vi "VDD.vi"(8 "error in (no error)":errorcluster, 10 "Multimetru":refnum<visa-resource-name>="GPIB0::24::INSTR", 11 "SMU":refnum<visa-resource-name>="GPIB0::1::INSTR") -> (0 "error out":errorcluster, 1 "Histeresis":dbl, 2 "VDD_min_down":dbl, 3 "VDD_min_up":dbl)   [LabVIEW 2020]
uses:
  76adbe7d-9721-415f-b48f-f6746734e94a.vi
  a5dc711f-f3d3-4f32-829f-27d9f17150a9.vi
  eb78ffcd-5ce8-4557-ad43-e495a85b1885.vi
  a097896c-11b6-4113-a8a2-d510a1bfe5c9.vi
  204cda9c-a345-42f7-b798-14036ec7fdcd.vi
  845bcc2d-13a0-4ca5-84b0-81bd2e2c0ef6.vi
  9402af0b-bcf9-4b6a-9b28-d1ed00ce5349.vi
  <vilib>/Analysis/1siggen.llb/Ramp Pattern by Delta.vi
  Drivers/agilent_3446x_series/Agilent 3446X Series/Public/Data/Read (Single Point).vi
  Drivers/keithley_2450/Keithley 2450/Keithley 2450.lvlib
  Drivers/agilent_3446x_series/Agilent 3446X Series/Agilent 3446X Series.lvlib
  <vilib>/Analysis/NI_AALBase.lvlib
panel:
  in  "Tab Control":enum32{"Page 1", "Page 2"}(tab)
  out "IDD up":dbl
  out "noOfDevs out":u32=1
  out "VDD curent up":dbl
  out "VDD curent down":dbl
  out "noOfDevs out 2":u32=1
  out "IDD down":dbl
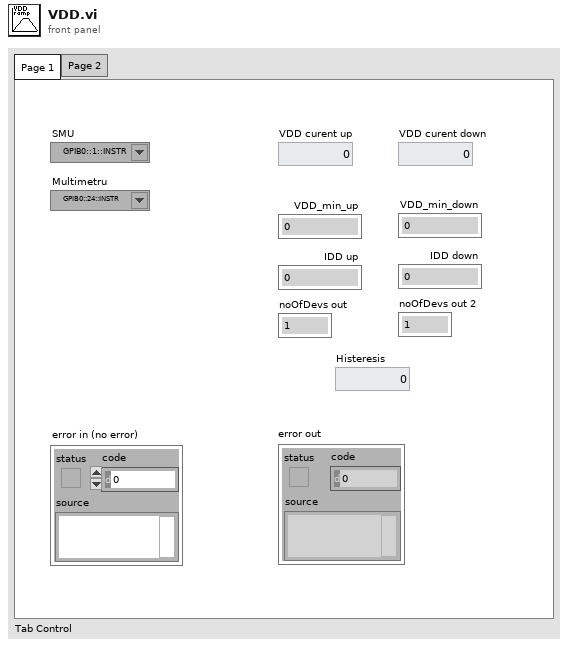
[diagram p1: front panel]
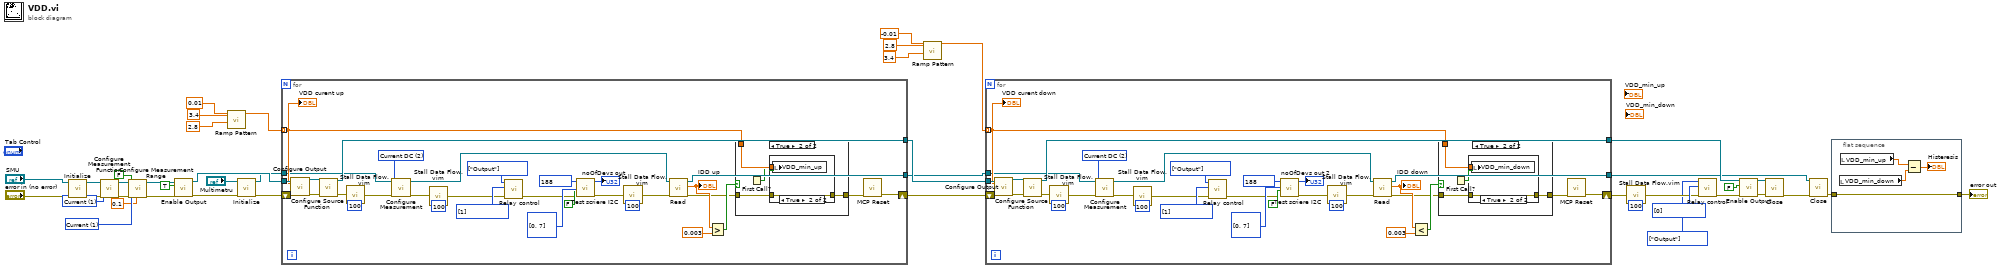
[diagram p0: block diagram]
diagram:
  w25 = u16 1 items=["Volts", "Current", "Resistance"] ("Function (0: Volts)")
  w26 = u16 1 items=["Volts", "Current", "Auto Resistance", "Manual Resistance", "Digitize Voltage", "Digitize Current"] ("Function (0: Volts)")
  w33 = enum8{"Output", "Input", "Unchange"}[] [enum."Output"] items=["Output", "Input", "Unchange"] ("gpioDir")
  w35 = u16[] [0] items=["low"=0, "high"=1, "Unchange"=255] ("outputValues")
  n1 = call "Initialize.vi"("error in (no error)"="error in (no error)", "VISA resource name"="SMU") -> ("error out"=w30:errorcluster, "VISA resource name out"=w31:refnum<visa-resource-name>)  [unwired: 8 in]
  n2 = call "Configure Measurement Function.vi"("error in (no error)"=w30, "Function (0: Volts)"=w26, "VISA resource name"=w31) -> ("error out"=w28:errorcluster, "VISA resource name out"=w29:refnum<visa-resource-name>)  [unwired: 7 in]
  n3 = call "Configure Measurement Range.vi"("Manual Range (1.0)"=0.1, "error in (no error)"=w28, "Enable Auto Range (T:Enable)"=FALSE, "Function (0: Volts)"=w25, "VISA resource name"=w29) -> ("error out"=w23:errorcluster, "VISA resource name out"=w22:refnum<visa-resource-name>)  [unwired: 5 in]
  n4 = call "Enable Output.vi"("error in (no error)"=w23, "Enable Output (T: Enable)"=TRUE, "VISA resource name"=w22) -> ("error out"=w16:errorcluster, "VISA resource name out"=w14:refnum<visa-resource-name>)  [unwired: 7 in]
  n5 = call-poly <vilib>:"Ramp Pattern.vi"("start"=2.8, "end"=3.4, "delta"=0.01) -> ("Ramp Pattern"=w18:dbl[])  [unwired: 6 in, 2 out]
  n6 = call "Initialize.vi"("error in (no error)"=w16, "VISA resource name"="Multimetru") -> ("error out"=w15:errorcluster, "VISA resource name out"=w13:refnum<visa-resource-name>)  [unwired: 8 in]
  n7 = for {
    tunnel: [w72] -> w7
    shift-right: [w44] -> w9
    shift-left: w15 -> [w55]
    tunnel: w14 -> [w56]
    tunnel: [w53] -> w8
    tunnel: w18 -> [w48] mode=indexing
    tunnel: w13 -> [w46]
    w68 = u16[] [1] items=["low"=0, "high"=1, "Unchange"=255] ("outputValues")
    w69 = enum8{"Output", "Input", "Unchange"}[] [enum."Output"] items=["Output", "Input", "Unchange"] ("gpioDir")
    w75 = 2 items=["Continuity", "Current AC", "Current DC", "Diode", "Frequency", "Resistance 4-wire", "Period", "Resistance 2-wire", "Temperature", "Voltage AC", "Voltage DC", "Voltage DC Ratio", "Capacitance"] ("Measurement Function (10: Voltage DC)")
    n8 = call "Configure Output.vi"("VISA resource name"=w56, "Source Level (0)"=w48, "error in (no error)"=w55) -> ("VISA resource name out"=w58:refnum<visa-resource-name>, "error out"=w57:errorcluster)  [unwired: 11 in]
    n9 = call "Configure Source Function.vi"("error in (no error)"=w57, "VISA resource name"=w58) -> ("error out"=w54:errorcluster, "VISA resource name out"=w53:refnum<visa-resource-name>)  [unwired: 8 in]
    n10 = call "Stall Data Flow.vim"("value in"=w54, "milliseconds to wait"=u32 100) -> ("value out"=w47:errorcluster)  [unwired: 1 out]
    n11 = call "Configure Measurement.vi"("error in (no error)"=w47, "Measurement Function (10: Voltage DC)"=w75, "VISA resource name"=w46) -> ("error out"=w67:errorcluster, "VISA resource name out"=w66:refnum<visa-resource-name>)  [unwired: 7 in]
    n12 = call "Stall Data Flow.vim"("value in"=w67, "milliseconds to wait"=u32 100) -> ("value out"=w60:errorcluster)  [unwired: 1 out]
    n13 = call "Relay control.vi"("error in (no error) 2"=w60, "outputValues"=w68, "gpioDir"=w69) -> ("error out"=w59:errorcluster)  [unwired: 8 in]
    n14 = call "Test scriere I2C.vi"("error in (no error)"=w59, "use7bitAddress"=FALSE, "i2cTxData"=u8[] [0, 7], "slaveAddress"=u8 188) -> ("error out"=w61:errorcluster, "noOfDevs out"=→"noOfDevs out":u32)  [unwired: 5 in, 1 out]
    n15 = call "Stall Data Flow.vim"("value in"=w61, "milliseconds to wait"=u32 100) -> ("value out"=w73:errorcluster)  [unwired: 1 out]
    n16 = call-poly "Read.vi"("error in (no error)"=w73, "VISA resource name"=w66) -> ("error out"=w49:errorcluster, "Measurement"=w52:dbl, "VISA resource name out"=w72:refnum<visa-resource-name>)  [unwired: 7 in]
    "IDD up" <- w52
    n17 = Greater?(x=w52, y=0.003) -> (0:w50:bool)
    n18 = case shown="True" w50 {
      tunnel: w49 -> [w76 w78]
      tunnel: [w76 w77] -> w45
      tunnel: w48 -> [_ w80]
      frame False {
      }
      frame True {
        n19 = First Call?() -> (First Call?: T/F=w79:bool)
        n20 = case shown="True" w79 {
          tunnel: w80 -> [_ w83]
          tunnel: w78 -> [w81 w82]
          tunnel: [w81 w82] -> w77
          frame False {
          }
          frame True {
            n21 = local write "VDD_min_up"(w83) -> ()
          }
        }
      }
    }
    n22 = call "MCP Reset.vi"("error in (no error)"=w45) -> ("error out"=w44:errorcluster)  [unwired: 10 in]
    "VDD curent up" <- w48
  }
  n23 = call-poly <vilib>:"Ramp Pattern.vi"("start"=3.4, "end"=2.8, "delta"=-0.01) -> ("Ramp Pattern"=w6:dbl[])  [unwired: 6 in, 2 out]
  n24 = for {
    tunnel: [w112] -> w3
    shift-right: [w84] -> w5
    shift-left: w9 -> [w95]
    tunnel: w8 -> [w96]
    tunnel: [w93] -> w4
    tunnel: w6 -> [w88] mode=indexing
    tunnel: w7 -> [w86]
    w108 = u16[] [1] items=["low"=0, "high"=1, "Unchange"=255] ("outputValues")
    w109 = enum8{"Output", "Input", "Unchange"}[] [enum."Output"] items=["Output", "Input", "Unchange"] ("gpioDir")
    w115 = 2 items=["Continuity", "Current AC", "Current DC", "Diode", "Frequency", "Resistance 4-wire", "Period", "Resistance 2-wire", "Temperature", "Voltage AC", "Voltage DC", "Voltage DC Ratio", "Capacitance"] ("Measurement Function (10: Voltage DC)")
    n25 = call "Configure Output.vi"("VISA resource name"=w96, "Source Level (0)"=w88, "error in (no error)"=w95) -> ("VISA resource name out"=w98:refnum<visa-resource-name>, "error out"=w97:errorcluster)  [unwired: 11 in]
    n26 = call "Configure Source Function.vi"("error in (no error)"=w97, "VISA resource name"=w98) -> ("error out"=w94:errorcluster, "VISA resource name out"=w93:refnum<visa-resource-name>)  [unwired: 8 in]
    n27 = call "Stall Data Flow.vim"("value in"=w94, "milliseconds to wait"=u32 100) -> ("value out"=w87:errorcluster)  [unwired: 1 out]
    n28 = call "Configure Measurement.vi"("error in (no error)"=w87, "Measurement Function (10: Voltage DC)"=w115, "VISA resource name"=w86) -> ("error out"=w107:errorcluster, "VISA resource name out"=w106:refnum<visa-resource-name>)  [unwired: 7 in]
    n29 = call "Stall Data Flow.vim"("value in"=w107, "milliseconds to wait"=u32 100) -> ("value out"=w100:errorcluster)  [unwired: 1 out]
    n30 = call "Relay control.vi"("error in (no error) 2"=w100, "outputValues"=w108, "gpioDir"=w109) -> ("error out"=w99:errorcluster)  [unwired: 8 in]
    n31 = call "Test scriere I2C.vi"("error in (no error)"=w99, "use7bitAddress"=FALSE, "i2cTxData"=u8[] [0, 7], "slaveAddress"=u8 188) -> ("error out"=w101:errorcluster, "noOfDevs out"=→"noOfDevs out 2":u32)  [unwired: 5 in, 1 out]
    n32 = call "Stall Data Flow.vim"("value in"=w101, "milliseconds to wait"=u32 100) -> ("value out"=w113:errorcluster)  [unwired: 1 out]
    n33 = call-poly "Read.vi"("error in (no error)"=w113, "VISA resource name"=w106) -> ("error out"=w89:errorcluster, "Measurement"=w92:dbl, "VISA resource name out"=w112:refnum<visa-resource-name>)  [unwired: 7 in]
    "IDD down" <- w92
    n34 = Less?(x=w92, y=0.003) -> (x < y?=w90:bool)
    n35 = case shown="True" w90 {
      tunnel: w89 -> [w116 w118]
      tunnel: [w116 w117] -> w85
      tunnel: w88 -> [_ w120]
      frame False {
      }
      frame True {
        n36 = First Call?() -> (First Call?: T/F=w119:bool)
        n37 = case shown="True" w119 {
          tunnel: w120 -> [_ w123]
          tunnel: w118 -> [w121 w122]
          tunnel: [w121 w122] -> w117
          frame False {
          }
          frame True {
            n38 = local write "VDD_min_down"(w123) -> ()
          }
        }
      }
    }
    n39 = call "MCP Reset.vi"("error in (no error)"=w85) -> ("error out"=w84:errorcluster)  [unwired: 10 in]
    "VDD curent down" <- w88
  }
  n40 = call "Stall Data Flow.vim"("value in"=w5, "milliseconds to wait"=u32 100) -> ("value out"=w34:errorcluster)  [unwired: 1 out]
  n41 = call "Relay control.vi"("error in (no error) 2"=w34, "outputValues"=w35, "gpioDir"=w33) -> ("error out"=w32:errorcluster)  [unwired: 8 in]
  n42 = call "Enable Output.vi"("error in (no error)"=w32, "Enable Output (T: Enable)"=FALSE, "VISA resource name"=w4) -> ("error out"=w38:errorcluster, "VISA resource name out"=w39:refnum<visa-resource-name>)  [unwired: 7 in]
  n43 = call "Close.vi"("error in (no error)"=w38, "VISA resource name"=w39) -> ("error out"=w37:errorcluster)  [unwired: 9 in]
  n44 = call "Close.vi"("error in (no error)"=w37, "VISA resource name"=w3) -> ("error out"=w1:errorcluster)  [unwired: 9 in]
  n45 = flat-sequence {
    tunnel: [w127] -> w2
    tunnel: w1 -> [w127]
    frame #0 {
      n46 = local read "VDD_min_down"() -> (w125:dbl)
      n47 = local read "VDD_min_up"() -> (w126:dbl)
      n48 = Subtract(x=w126, y=w125) -> (x-y=→"Histeresis":dbl)
    }
  }
  "error out" <- w2
